vi "Reverse backwards past comma.vi"(7 "JSON":string, 9 "Offset":i32) -> (1 "Offset of first non-whitespace":i32, 3 "Parser State":T1)   [LabVIEW 2015, in "JSONtext.lvlib"]
uses:
  JSONtext.lvlib
  Parsing State.ctl
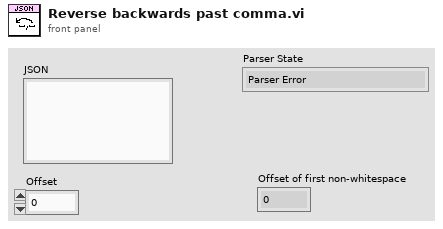
[diagram p1: front panel]
types:
  T1 = typedef "JSONtext.lvlib/Parsing State.ctl" = enum16{"Parser Error", "Object", "Array", "String", "Number/Other", "Leading Whitespace", "Object end", "Array end", "Value end"}
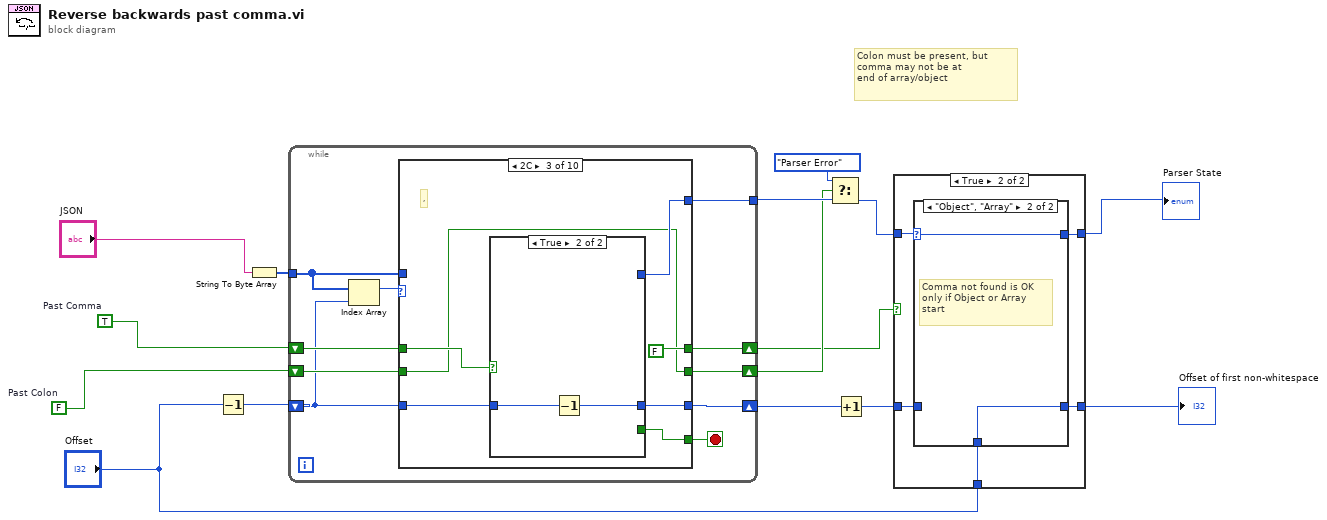
[diagram p0: block diagram]
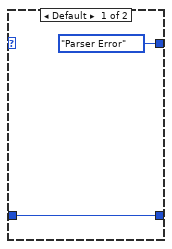
[diagram p3: hidden frame]
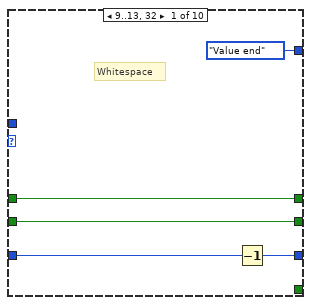
[diagram p4: hidden frame]
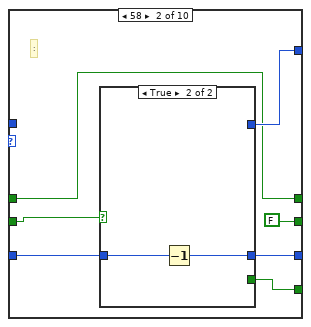
[diagram p5: hidden frame]
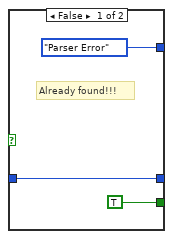
[diagram p6: hidden frame]
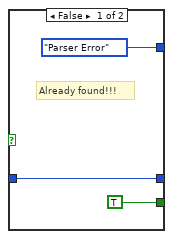
[diagram p7: hidden frame]
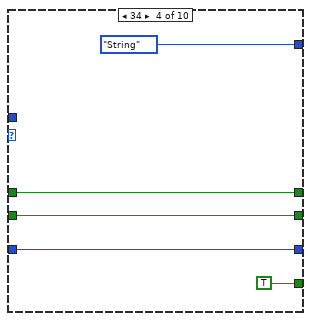
[diagram p8: hidden frame]
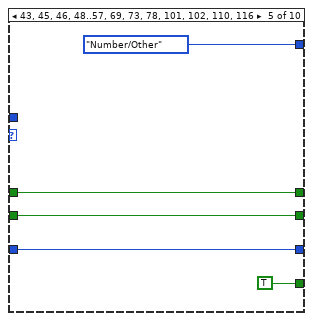
[diagram p9: hidden frame]
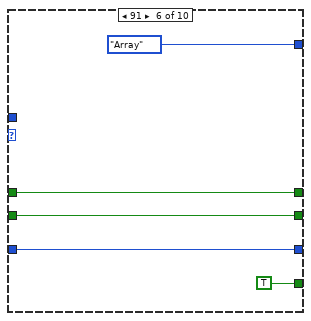
[diagram p10: hidden frame]
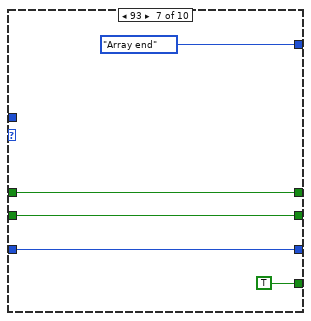
[diagram p11: hidden frame]
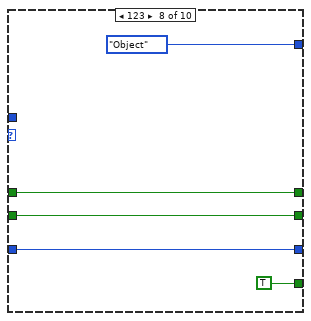
[diagram p12: hidden frame]
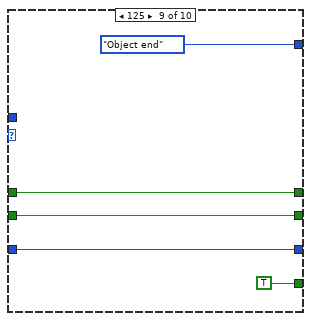
[diagram p13: hidden frame]
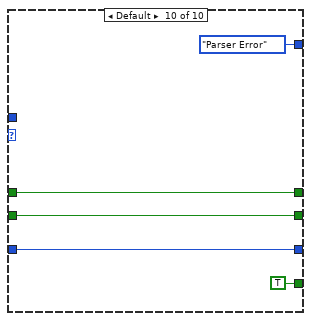
[diagram p14: hidden frame]
diagram:
  w12 = FALSE  # Past Colon
  w13 = TRUE  # Past Comma
  # "Colon must be present, but\ncomma may not be at\nend of array/object"
  n1 = Decrement(x="Offset") -> (x-1=w2:i32)
  n2 = String To Byte Array(string="JSON") -> (unsigned byte array=w11:u8[])
  n3 = while {
    tunnel: w11 -> [w24]
    shift-right: [w21] -> w4
    shift-left: w2 -> [w16]
    tunnel: [w23] -> w10
    shift-right: [w20] -> w7
    shift-left: w13 -> [w19]
    shift-right: [w17] -> w8
    shift-left: w12 -> [w18]
    stop <- w22 stop-if-true
    n4 = Index Array(array=w24, index=w16) -> (element=w25:u8)
    n5 = case shown="2C" w25 {
      tunnel: w24 -> [_ _ _ _ _ _ _ _ _ _]
      tunnel: [Parsing_State."Value end" w35 w47 Parsing_State."String" Parsing_State."Number/Other" Parsing_State."Array" Parsing_State."Array end" Parsing_State."Object" Parsing_State."Object end" Parsing_State."Parser Error"] -> w23
      tunnel: [_ w34 w46 TRUE TRUE TRUE TRUE TRUE TRUE TRUE] -> w22
      tunnel: w16 -> [w30 w37 w49 w57 w62 w67 w72 w77 w82 w89]
      tunnel: [w29 w36 w48 w57 w62 w67 w72 w77 w82 w89] -> w21
      tunnel: [w27 w31 FALSE ("Allow Comma") w56 w61 w66 w71 w76 w81 w86] -> w20
      tunnel: w19 -> [w27 w31 w45 w56 w61 w66 w71 w76 w81 w86]
      tunnel: [w26 FALSE ("Allow Comma") w43 w55 w60 w65 w70 w75 w80 w85] -> w17
      tunnel: w18 -> [w26 w33 w43 w55 w60 w65 w70 w75 w80 w85]
      frame 9..13, 32 {
        # "Whitespace"
        n6 = Decrement(x=w30) -> (x-1=w29:i32)
      }
      frame 58 {
        # ":"
        n7 = case shown="True" w33 {
          tunnel: w37 -> [w39 w42]
          tunnel: [w39 w41] -> w36
          tunnel: [Parsing_State."Parser Error" _] -> w35
          tunnel: [TRUE _] -> w34
          frame False {
            # "Already found!!!"
          }
          frame True {
            n8 = Decrement(x=w42) -> (x-1=w41:i32)
          }
        }
      }
      frame 44 {
        # ","
        n9 = case shown="True" w45 {
          tunnel: w49 -> [w51 w54]
          tunnel: [w51 w53] -> w48
          tunnel: [Parsing_State."Parser Error" _] -> w47
          tunnel: [TRUE _] -> w46
          frame False {
            # "Already found!!!"
          }
          frame True {
            n10 = Decrement(x=w54) -> (x-1=w53:i32)
          }
        }
      }
      frame 34 {
      }
      frame 43, 45, 46, 48..57, 69, 73, 78, 101, 102, 110, 116 {
      }
      frame 91 {
      }
      frame 93 {
      }
      frame 123 {
      }
      frame 125 {
      }
      frame Default {
      }
    }
  }
  n11 = Select(t=Parsing_State."Parser Error", s=w8, f=w10) -> (s? t:f=w6:T1)
  n12 = Increment(x=w4) -> (x+1=w1:i32)
  n13 = case shown="True" w7 {
    tunnel: w6 -> [w91 w96]
    tunnel: [w91 w95] -> w15
    tunnel: [w90 w94] -> w5
    tunnel: w1 -> [w90 w92]
    tunnel: "Offset" -> [_ w93]
    frame False {
    }
    frame True {
      n14 = case shown="\"Object\", \"Array\"" w96 {
        selector: w96 -> [_ w100]
        tunnel: [Parsing_State."Parser Error" w100] -> w95
        tunnel: [w97 w99] -> w94
        tunnel: w93 -> [_ w99]
        tunnel: w92 -> [w97 _]
        frame Default {
        }
        frame "Object", "Array" {
          # "Comma not found is OK\nonly if Object or Array\nstart"
        }
      }
    }
  }
  "Parser State" <- w15
  "Offset of first non-whitespace" <- w5
